vi "DSF.Engine.Interface.Get Response FIFO.vi"(11 "Interface in":refnum<class "DSF.Engine.Interface.lvclass">) -> (2 "Response FIFO":T1, 3 "Interface out":refnum<class "DSF.Engine.Interface.lvclass">)   [LabVIEW 2016, in "DSF.Engine.lvlib" / "DSF.Engine.Interface.lvclass"]
uses:
  DSF.Engine.Interface.lvclass
  DSF.Engine.Interface.RT FIFO.Data.16B.ctl
  DSF.Engine.Interface.RT FIFO.Ref.16B.ctl
  DSF.Engine.Interface.RT FIFO.Payload.16B.ctl
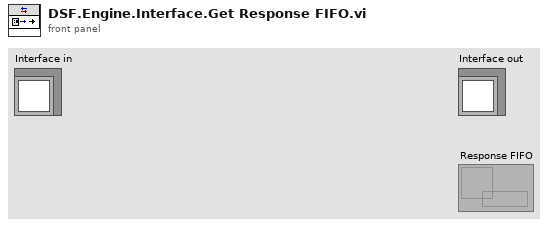
[diagram p1: front panel]
types:
  T1 = typedef "DSF.Engine.lvlib/DSF.Engine.Interface.lvclass/DSF.Engine.Interface.RT FIFO.Ref.16B.ctl" = refnum<k33>
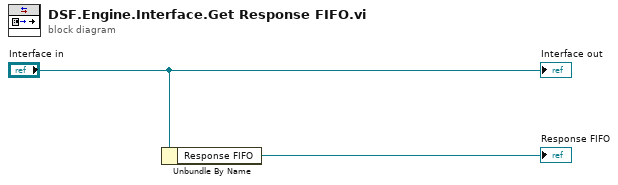
[diagram p0: block diagram]
diagram:
  n1 = Unbundle By Name("Interface in") -> ("Response FIFO"=→"Response FIFO":T1)
  "Interface out" <- "Interface in"
